vi "updateSpecINFO.vi"(11 "specInfo":T1 {"Charge [pC]" format="%0.4f"}) -> ()   [LabVIEW 2011, in "MagAnalysis_Online.lvclass"]
uses:
  MagAnalysis_Online.lvclass
  specInfo_TypDef.ctl
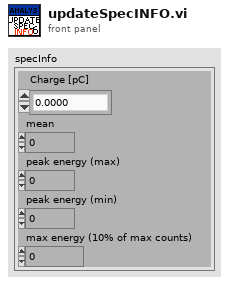
[diagram p1: front panel]
types:
  T1 = typedef "specInfo_TypDef.ctl" = cluster{"Charge [pC]":dbl, "mean":dbl, "peak energy (max)":dbl, "peak energy (min)":dbl, "max energy (10% of max counts)":dbl}
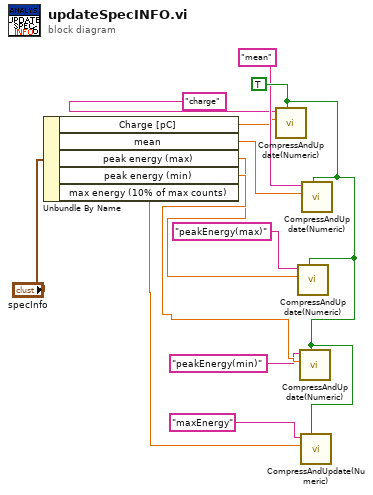
[diagram p0: block diagram]
diagram:
  w12 = TRUE ("force CVT update (false)")
  n1 = Unbundle By Name("specInfo") -> ("Charge [pC]"=w3:dbl, "mean"=w4:dbl, "peak energy (max)"=w7:dbl, "peak energy (min)"=w9:dbl, "max energy (10% of max counts)"=w10:dbl)
  n2 = call "CompressAndUpdate(Numeric).vi"("force CVT update (false)"=w12, "Numeric"=w3, "command or variable name"="charge") -> ()  [unwired: 8 in, 1 out]
  n3 = call "CompressAndUpdate(Numeric).vi"("force CVT update (false)"=w12, "Numeric"=w7, "command or variable name"="peakEnergy(max)") -> ()  [unwired: 8 in, 1 out]
  n4 = call "CompressAndUpdate(Numeric).vi"("force CVT update (false)"=w12, "Numeric"=w9, "command or variable name"="peakEnergy(min)") -> ()  [unwired: 8 in, 1 out]
  n5 = call "CompressAndUpdate(Numeric).vi"("force CVT update (false)"=w12, "Numeric"=w10, "command or variable name"="maxEnergy") -> ()  [unwired: 8 in, 1 out]
  n6 = call "CompressAndUpdate(Numeric).vi"("force CVT update (false)"=w12, "Numeric"=w4, "command or variable name"="mean") -> ()  [unwired: 8 in, 1 out]
